vi "Test Roundtrip Serialize Fixed Length Data Types.vi"(8 "error in (no error)":errorcluster) -> (0 "error out":errorcluster)   [LabVIEW 2013]
uses:
  <vilib>/addons/_JKI Toolkits/Caraya/classes/Test/Test.lvclass
  <vilib>/addons/_JKI Toolkits/Caraya/classes/Assert/Assert.lvclass
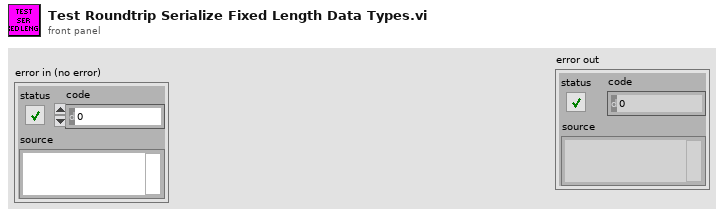
[diagram p1: front panel]
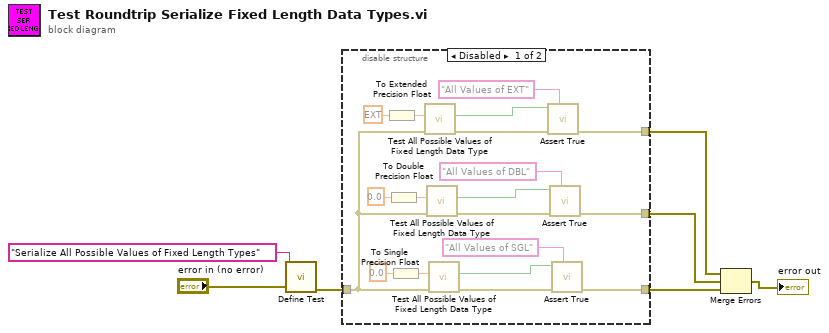
[diagram p0: block diagram]
diagram:
  n1 = call <vilib>:"Define Test.vi"("error in (no error)"="error in (no error)", "Label (VI Title)"="Serialize All Possible Values of Fixed Length Types") -> ("error out"=w2:errorcluster)  [unwired: 9 in]
  n2 = disable-structure shown="Disabled" {
    disable-tunnel: [w26 _] -> w4
    disable-tunnel: [w17 _] -> w3
    disable-tunnel: w2 -> [w12 _]
    disable-tunnel: [w11 _] -> w1
    frame Disabled {
      n3 = To Extended Precision Float(1:ext 0.0) -> (0:w15:ext)
      n4 = To Double Precision Float(number=0.0) -> (double precision float=w19:dbl)
      n5 = To Single Precision Float(number=sgl 0.0) -> (single precision float=w24:sgl)
      n6 = call "Test All Possible Values of Fixed Length Data Type.vi"("error in"=w12, "Fixed Length Data In"=w15) -> ("error out"=w14:errorcluster, "Pass?"=w8:bool)  [unwired: 7 in, 1 out]
      n7 = call "Test All Possible Values of Fixed Length Data Type.vi"("error in"=w12, "Fixed Length Data In"=w19) -> ("error out"=w20:errorcluster, "Pass?"=w9:bool)  [unwired: 7 in, 1 out]
      n8 = call "Test All Possible Values of Fixed Length Data Type.vi"("error in"=w12, "Fixed Length Data In"=w24) -> ("error out"=w23:errorcluster, "Pass?"=w10:bool)  [unwired: 7 in, 1 out]
      n9 = call <vilib>:"Assert True.vi"("Label"="All Values of EXT", "error in (no error)"=w14, "True?"=w8) -> ("error out"=w11:errorcluster)  [unwired: 8 in]
      n10 = call <vilib>:"Assert True.vi"("Label"="All Values of DBL", "error in (no error)"=w20, "True?"=w9) -> ("error out"=w17:errorcluster)  [unwired: 8 in]
      n11 = call <vilib>:"Assert True.vi"("Label"="All Values of SGL", "error in (no error)"=w23, "True?"=w10) -> ("error out"=w26:errorcluster)  [unwired: 8 in]
    }
    frame Enabled {
    }
  }
  n12 = Merge Errors(w1, w3, w4) -> (→"error out":errorcluster)
